vi "Simple.vi"() -> ()   [LabVIEW 2018]
doc: "Demonstrates compiling a logic-free mustache template string. Only variable tags are used in this example."
uses:
  Toolkit/Support/Compile with String Array.vi
  Toolkit/Toolkit.lvlib
panel:
  in  "Data":cluster{"Key":string, "Value":string}[](array[cluster])=[{"Key"="greeting", "Value"="Hello"}, {"Key"="name", "Value"="World"}]
  out "Output":string
  in  "Input":string="This is a simple mustache template.\n\n{{greeting}} {{name}}!\n\nAny kind of text, or string, can be created as a mustache template, but it is particularly useful for creating HTML files."
  # "Overview: Demonstrates compiling a mustache template string with only variable tags\nInstructions:\n1. Run this VI"
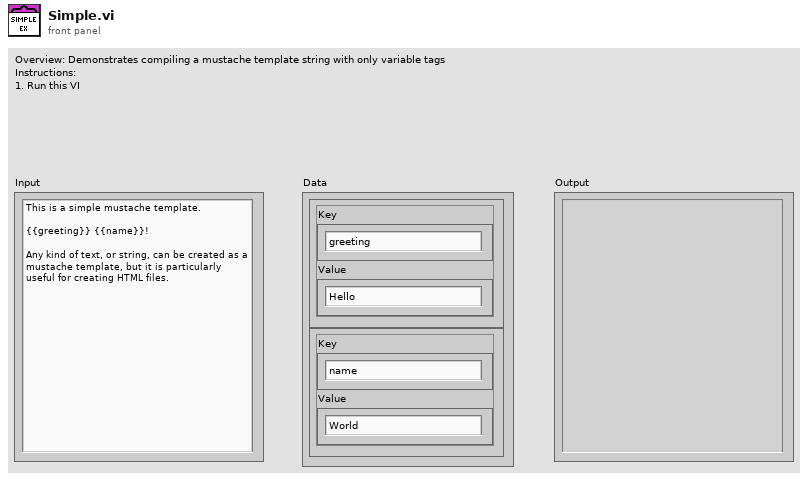
[diagram p1: front panel]
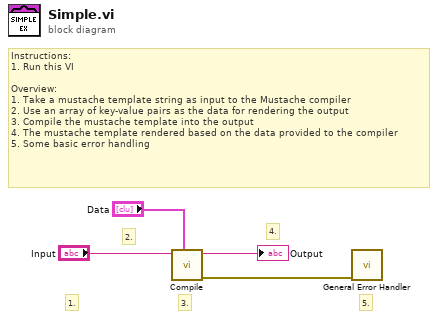
[diagram p0: block diagram]
diagram:
  # "5."
  # "4."
  # "3."
  # "2."
  # "1."
  # "Instructions:\n1. Run this VI\n\nOverview:\n1. Take a mustache template string as input to the Mustache compiler\n2. Use an array of key-value pairs as the data for rendering the output\n3. Compile the mustache template into the output\n4. The mustache template rendered based on the data provided to the compiler\n5. Some basic error handling"
  n1 = call-poly "Compile.vi"("Data"="Data", "Input"="Input") -> ("Error Out"=w4:errorcluster, "Output"=→"Output":string)  [unwired: 8 in]
  n2 = call <vilib>:"General Error Handler.vi"("error in (no error)"=w4) -> ()  [unwired: 10 in, 5 out]
